vi "Set Root Hierarchy.vi"(8 "error in (no error)":errorcluster, 10 "Root Hierarchy":string[](array[string]), 11 "Config Storage in":refnum<class "Config Storage.lvclass">) -> (0 "error out":errorcluster, 3 "Config Storage out":refnum<class "Config Storage.lvclass">)   [LabVIEW 2020, in "CDM-Config.lvlib" / "Config Storage.lvclass"]
uses:
  Config Storage.lvclass
  Config Storage.lvclass/Config Storage.ctl
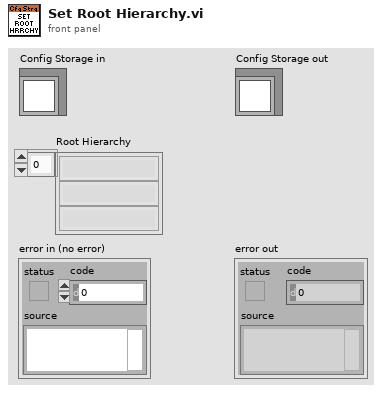
[diagram p1: front panel]
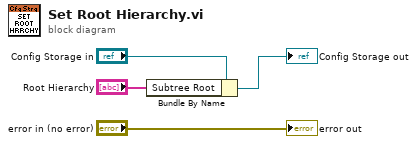
[diagram p0: block diagram]
diagram:
  n1 = Bundle By Name(cluster="Config Storage in", "Subtree Root"="Root Hierarchy") -> (→"Config Storage out":refnum<class "Config Storage.lvclass">)
  "error out" <- "error in (no error)"
